vi "Pid_v13.vi"() -> ()   [LabVIEW 2020]
panel:
  out "u - Comanda":dbl(graph)=49.999877814419186
  out "y - Iesirea":dbl(slide)=49.99941110945184 scale=40.0..60.0
  in  "stop":bool
  out "y":dbl=49.99941110945184
  out "u - Comanda":dbl(slide)=49.999877814419186 scale=40.0..60.0
  out "y,r,u":cluster{"r-Set point":dbl, dbl, dbl}(graph)={"r-Set point"=49.99941110945184, 50.0, 49.999877814419186}
  in  "Kd":dbl(slide)=0.1111111111111111 scale=0.0..0.5
  in  "Kp":dbl(slide)=0.3508771929824561 scale=0.0..2.5
  in  "Ki":dbl(slide)=0.8888888888888888 scale=0.0..2.0
  in  "r - Set point":dbl(slide)=50.0 scale=40.0..60.0
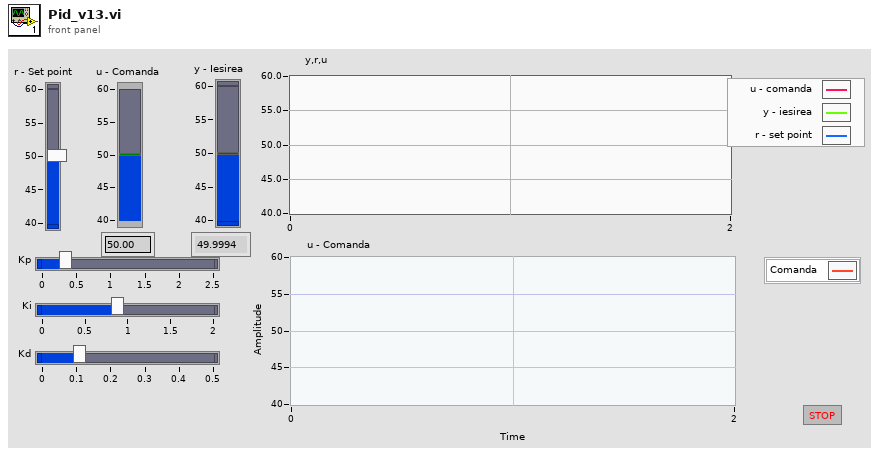
[diagram p1: front panel]
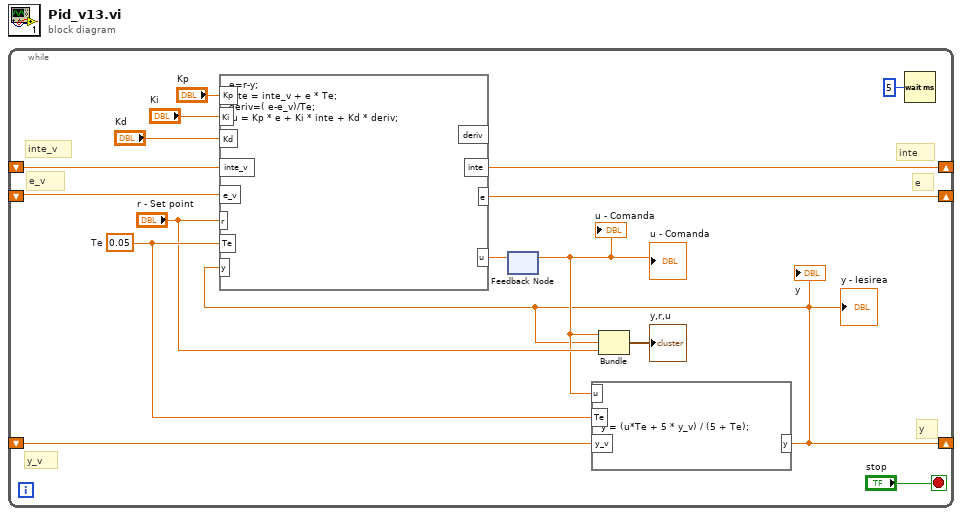
[diagram p0: block diagram]
diagram:
  n1 = while {
    shift-right: [w7] -> _
    shift-left: _ -> [w12]
    shift-right: [w2] -> _
    shift-left: _ -> [w6]
    shift-right: [w13] -> _
    shift-left: _ -> [w14]
    stop <- "stop" stop-if-true
    w5 = 0.05  # Te
    # "e_v"
    # "e"
    # "inte_v"
    # "inte"
    # "y_v"
    # "y"
    n2 = feedback #1() -> (w3:dbl)  [unwired: 1 in]
    "u - Comanda" <- w3
    "u - Comanda" <- w3
    n3 = formula code="y = (u*Te + 5 * y_v) / (5 + Te);"("y_v"=w6, "u"=w3, "Te"=w5) -> ("y"=w2:dbl)
    "y" <- w2
    "y - Iesirea" <- w2
    n4 = formula code="e=r-y;\ninte = inte_v + e * Te;\nderiv=( e-e_v)/Te;\n u = Kp * e + Ki * inte + Kd * deriv;"("inte_v"=w14, "Te"=w5, "e_v"=w12, "Kp"="Kp", "Ki"="Ki", "Kd"="Kd", "r"="r - Set point", "y"=w2) -> ("inte"=w13:dbl, "u"=w8:dbl, "e"=w7:dbl)  [unwired: 1 out]
    n5 = feedback-in #1(w8) -> ()
    n6 = Bundle("u"=w3, "y"=w2, "r - Set point"="r - Set point") -> (→"y,r,u":cluster{"u":dbl, "y":dbl, "r - Set point":dbl})  [unwired: 1 in]
    n7 = Wait (ms)(milliseconds to wait=u32 5) -> ()  [unwired: 1 out]
  }
